vi "Open_KEITHLEY2470.vi"(8 "error in (no error)":errorcluster, 11 "KEITHLEY2470":refnum<visa-resource-name>) -> (0 "error out":errorcluster, 3 "VISA resource name out":refnum<visa-resource-name>)   [LabVIEW 2019]
uses:
  <instrlib>/Keithley 2450/Keithley 2450.lvlib
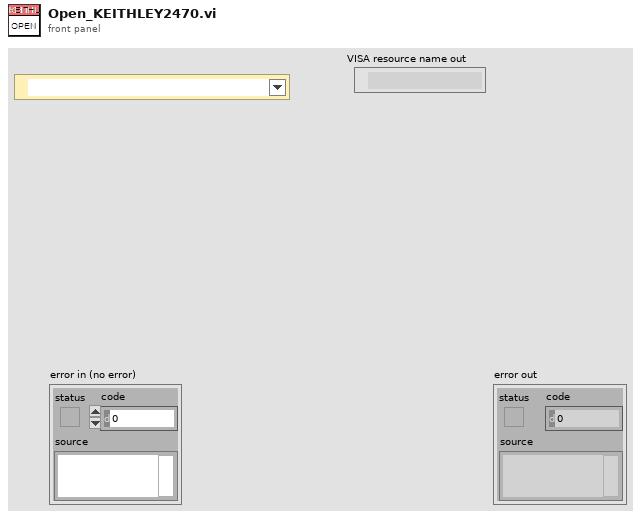
[diagram p1: front panel]
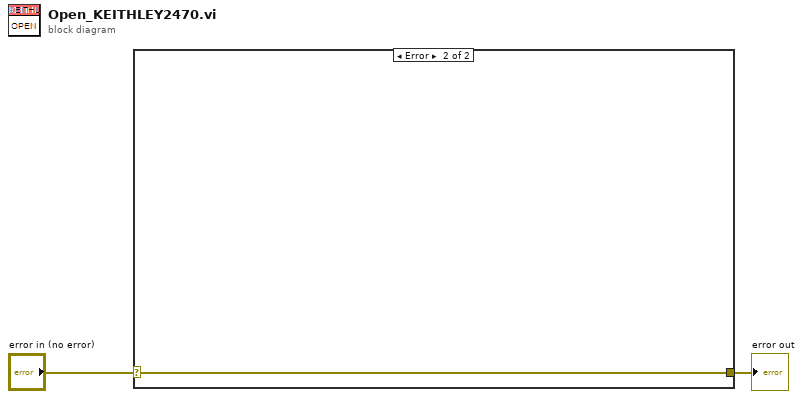
[diagram p0: block diagram]
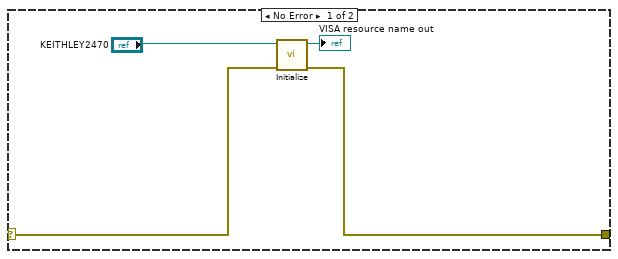
[diagram p2: hidden frame]
diagram:
  n1 = case shown="Error" "error in (no error)" {
    selector: "error in (no error)" -> [w6 w7]
    tunnel: [w5 w7] -> w1
    frame No Error {
      n2 = call <instrlib>:"Initialize.vi"("error in (no error)"=w6, "VISA resource name"="KEITHLEY2470") -> ("error out"=w5:errorcluster, "VISA resource name out"=→"VISA resource name out":refnum<visa-resource-name>)  [unwired: 8 in]
    }
    frame Error {
    }
  }
  "error out" <- w1
